vi "Edgertronic_CslcuateFillGraphic.vi"(3 "current # frames":dbl, 4 "Current Fill":i32, 5 "Current Settings:":T1={"Requested Genlock "="20140911165611", "Min Frame Clocks "="20140911165611", "Is Seq Clk Freq "="20140911165611", "Pretrigger Frames "="20140911165611", "Duration "="20140911165611", "Overclock "="20140911165611", "Requested Horizontal "="20140911165611", "Frames "="20140911165611", "Requested Pretrigger "="20140911165611", "Words per Frame "="20140911165611", "Buffer End "="20140911165611", "Clocks per Frame  "="20140911165611", "Requested Duration "="20140911165611", "Pretrigger "="20140911165611", "Post-trigger Frames "="20140911165611", "Vertical "="20140911165611", "Requested Vertical "="20140911165611", "Reqested Frame Rate "="20140911165611", "Frame Rate "="20140911165611", "Horizontal "="20140911165611", "Clocks per Exposure "="20140911165611", "Digital Gain "="20140911165611", "Exposure "="20140911165611", "Genlock "="20140911165611", "Analog Gain "="20140911165611", "Subsample "="20140911165611", "Requested Exposure "="20140911165611", "Iso "="20140911165611", "Requested Overclock "="20140911165611", "Requested Subsample "="20140911165611", "Requested Iso"="20140911165611", "Multishot"="20140911165611", "Requested Multishot"="20140911165611", "Monochrome"="20140911165611", "Requested mono"="20140911165611", "FPGA Temp"="20140911165611", "Is Temp"="20140911165611", "Posttrigger Duration"="20140911165611", "Pretrigger Duration"="20140911165611", "dacvrefadc"="20140911165611"}) -> (2 "Pretrigger Fill Level":cluster{u8, u8, u8}(slide)={100, 46, 32} scale=0.0..100.0)   [LabVIEW 2015]
uses:
  GET/SettingsCtrl.ctl
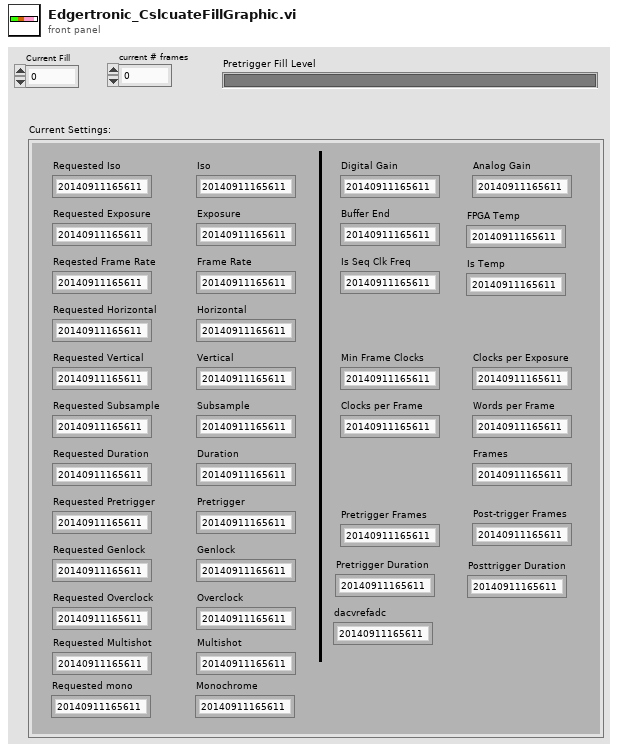
[diagram p1: front panel]
types:
  T1 = typedef "SettingsCtrl.ctl" = cluster{"Requested Genlock ":string, "Min Frame Clocks ":string, "Is Seq Clk Freq ":string, "Pretrigger Frames ":string, "Duration ":string, "Overclock ":string, "Requested Horizontal ":string, "Frames ":string, "Requested Pretrigger ":string, "Words per Frame ":string, "Buffer End ":string, "Clocks per Frame  ":string, "Requested Duration ":string, "Pretrigger ":string, "Post-trigger Frames ":string, "Vertical ":string, "Requested Vertical ":string, "Reqested Frame Rate ":string, "Frame Rate ":string, "Horizontal ":string, "Clocks per Exposure ":string, "Digital Gain ":string, "Exposure ":string, "Genlock ":string, "Analog Gain ":string, "Subsample ":string, "Requested Exposure ":string, "Iso ":string, "Requested Overclock ":string, "Requested Subsample ":string, "Requested Iso":string, "Multishot":string, "Requested Multishot":string, "Monochrome":string, "Requested mono":string, "FPGA Temp":string, "Is Temp":string, "Posttrigger Duration":string, "Pretrigger Duration":string, "dacvrefadc":string}
  T2 = cluster{"current fill":u8, "pre-trigger":u8, "trigger fill":u8}
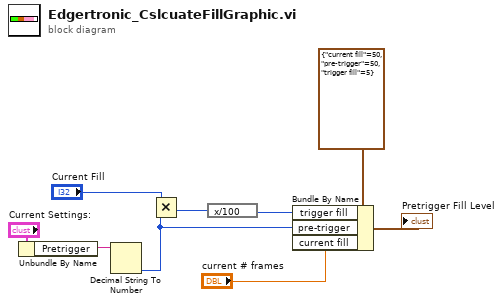
[diagram p0: block diagram]
diagram:
  n1 = Unbundle By Name("Current Settings:") -> ("Pretrigger"=w5:string)
  n2 = Decimal String To Number(string=w5) -> (number=w2:i32)  [unwired: 2 in, 1 out]
  n3 = Multiply(x="Current Fill", y=w2) -> (x*y=w8:i32)
  n4 = expression code="x/100"(w8) -> (w7:i32)
  n5 = Bundle By Name(cluster=T2 {"current fill"=50, "pre-trigger"=50, "trigger fill"=5} ("Pretrigger Fill Level"), "trigger fill"=w7, "pre-trigger"=w2, "current fill"="current # frames") -> (→"Pretrigger Fill Level":T2)
